vi "Test Rotate.vi"() -> ()   [LabVIEW 2017]
uses:
  Orient3d Class/Type Definitions/Quaternion.ctl
  <vilib>/Analysis/Matrix/Datatypes/RealMatrix.ctl
  <vilib>/Analysis/7linalg.llb/Real Transpose Matrix.vi
  Vec3d Class.lvclass
  Orient3d Class/Orient3d Class.lvclass
  <vilib>/Analysis/NI_AALPro.lvlib
  <vilib>/Analysis/Matrix/NI_Matrix.lvlib
panel:
  out "Quaternion 4":T1
  out "Quaternion 3":T1
  out "Quaternion 2":T1
  out "Rotated 2":cluster{"X":dbl, "Y":dbl, "Z":dbl}
  in  "Vector":cluster{"X":dbl, "Y":dbl, "Z":dbl}
  out "Rotation Matrix":T2
  in  "Quaternion":T1
  out "Rotated":cluster{"X":dbl, "Y":dbl, "Z":dbl}
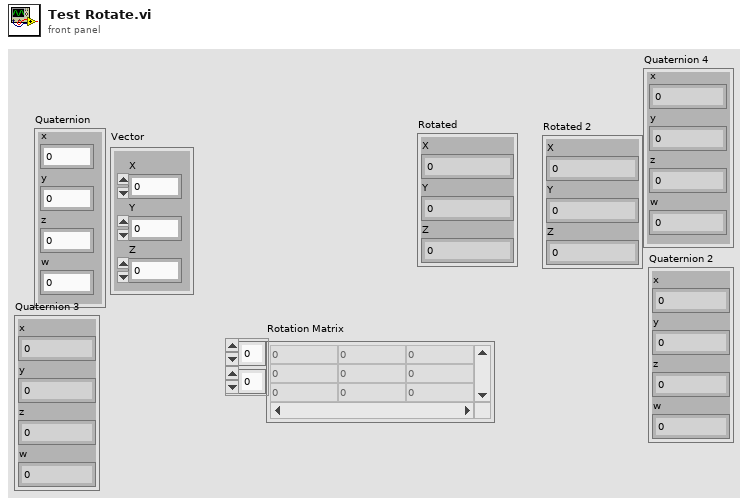
[diagram p1: front panel]
types:
  T1 = typedef "Quaternion.ctl" = cluster{"x":dbl, "y":dbl, "z":dbl, "w":dbl}
  T2 = typedef "NI_Matrix.lvlib/RealMatrix.ctl" = dbl[][]
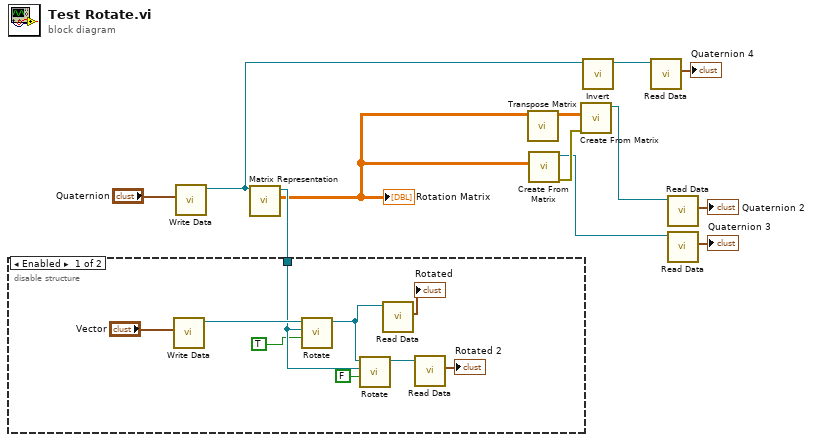
[diagram p0: block diagram]
diagram:
  n1 = call "Write Data.vi"("Quaternion"="Quaternion") -> ("Orient3d out"=w3:refnum<class "Orient3d Class.lvclass">)  [unwired: 9 in, 1 out]
  n2 = call "Matrix Representation.vi"("Orient3d in"=w3) -> ("Rotation Matrix"=w9:T2, "Orient3d out"=w11:refnum<class "Orient3d Class.lvclass">)  [unwired: 8 in, 1 out]
  "Rotation Matrix" <- w9
  n3 = disable-structure shown="Enabled" {
    disable-tunnel: w11 -> [w18 _]
    frame Enabled {
      n4 = call "Write Data.vi"("Data"="Vector") -> ("Vec3d Class out"=w19:refnum<class "Vec3d Class.lvclass">)  [unwired: 9 in, 1 out]
      n5 = call-dynamic "Rotate.vi"("Inverse?"=TRUE, "Orient3d in"=w18, "Vec3d in"=w19) -> ("Vec3d out"=w17:refnum<class "Vec3d Class.lvclass">)  [unwired: 7 in, 1 out]
      n6 = call-dynamic "Rotate.vi"("Inverse?"=FALSE, "Orient3d in"=w18, "Vec3d in"=w17) -> ("Vec3d out"=w15:refnum<class "Vec3d Class.lvclass">)  [unwired: 7 in, 1 out]
      n7 = call-dynamic "Read Data.vi"("Vec3d Class in"=w17) -> ("Data"=→"Rotated":cluster{"X":dbl, "Y":dbl, "Z":dbl})  [unwired: 8 in, 2 out]
      n8 = call-dynamic "Read Data.vi"("Vec3d Class in"=w15) -> ("Data"=→"Rotated 2":cluster{"X":dbl, "Y":dbl, "Z":dbl})  [unwired: 8 in, 2 out]
    }
    frame Disabled {
    }
  }
  n9 = call-poly <vilib>:"Transpose Matrix.vi"("Input Matrix"=w9) -> ("Matrix Transpose"=w8:T2)  [unwired: 9 in, 1 out]
  n10 = call "Create From Matrix.vi"("Rotation Matrix"=w9) -> ("error out"=w10:errorcluster, "Orient3d out"=w6:refnum<class "Orient3d Class.lvclass">)  [unwired: 9 in]
  n11 = call "Create From Matrix.vi"("error in"=w10, "Rotation Matrix"=w8) -> ("Orient3d out"=w7:refnum<class "Orient3d Class.lvclass">)  [unwired: 8 in, 1 out]
  n12 = call "Invert.vi"("Orient3d in"=w3) -> ("Orient3d out"=w2:refnum<class "Orient3d Class.lvclass">)  [unwired: 9 in, 1 out]
  n13 = call "Read Data.vi"("Orient3d in"=w2) -> ("Quaternion"=→"Quaternion 4":T1)  [unwired: 8 in, 2 out]
  n14 = call "Read Data.vi"("Orient3d in"=w7) -> ("Quaternion"=→"Quaternion 2":T1)  [unwired: 8 in, 2 out]
  n15 = call "Read Data.vi"("Orient3d in"=w6) -> ("Quaternion"=→"Quaternion 3":T1)  [unwired: 8 in, 2 out]
